vi "Pockels Cal load-Load handler.vi"(11 "Loaded pockels cal file":refnum<vi>) -> ()   [LabVIEW 2013]
uses:
  Typedefs/Which path.ctl
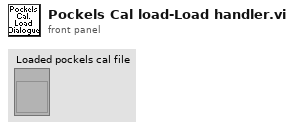
[diagram p1: front panel]
types:
  T1 = typedef "Which path.ctl" = enum16{"Configuration Files", "Calibration Files", "Images", "Setup.ini", "Loaded User profile.ini", "User's-Previous session.ini", "New user profile.ini", "Selected User profile.ini", "User profiles folder", "Power meter scaling.txt", "FOV Cal.ini"}
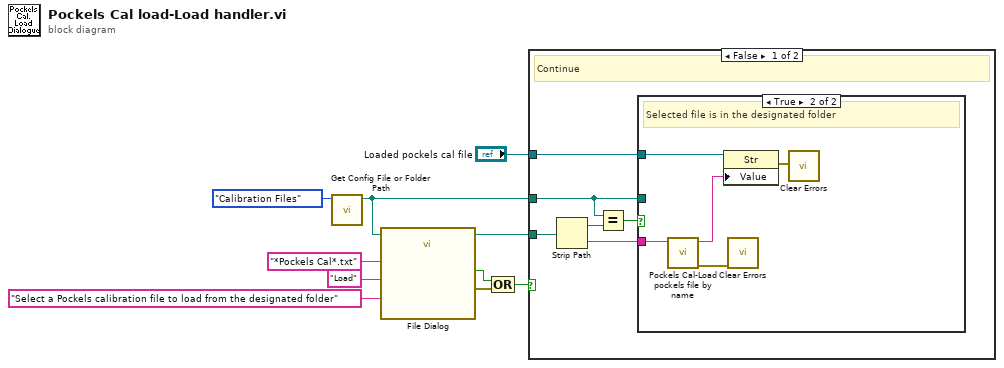
[diagram p0: block diagram]
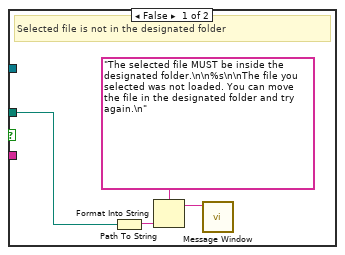
[diagram p2: hidden frame]
diagram:
  n1 = call "Get Config File or Folder Path.vi"("Which file or folder?"=Which_path."Calibration Files" ("Which file?")) -> ("File Path"=w2:path)  [unwired: 8 in, 2 out]
  n2 = call "File Dialog"("start path"=w2, "prompt"="Select a Pockels calibration file to load from the designated folder", "button label"="Load", "pattern (all files)"="*Pockels Cal*.txt") -> ("selected path"=w3:path, "cancelled"=w8:bool, "error out"=w7:errorcluster)  [unwired: 8 in, 1 out]
  n3 = Compound Arithmetic op=OR(w8, w7) -> (w6:bool)
  n4 = case shown="False" w6 {
    tunnel: w3 -> [w16 _]
    tunnel: w2 -> [w12 _]
    tunnel: "Loaded pockels cal file" -> [w11 _]
    frame False {
      # "Continue"
      n5 = Strip Path(path=w16) -> (stripped path=w14:path, name=w15:string)
      n6 = Equal?(x=w12, y=w14) -> (x = y?=w13:bool)
      n7 = case shown="True" w13 {
        tunnel: w15 -> [_ w24]
        tunnel: w12 -> [w17 _]
        tunnel: w11 -> [_ w25]
        frame False {
          # "Selected file is not in the designated folder"
          n8 = Path To String(path=w17) -> (string=w18:string)
          n9 = Format Into String(format string="The selected file MUST be inside the designated folder.\n\n%s\n\nThe file you selected was not loaded. You can move the file in the designated folder and try again.\n" ("Message string"), w18) -> (resulting string=w19:string)  [unwired: 2 in, 1 out]
          n10 = call "Message Window.vi"("Message string"=w19) -> ()  [unwired: 10 in, 1 out]
        }
        frame True {
          # "Selected file is in the designated folder"
          n11 = call "Pockels Cal-Load pockels file by name.vi"("Pockels cal file name"=w24) -> ("error out"=w21:errorcluster, "Pockels cal file name"=w23:string)  [unwired: 9 in]
          n12 = property class="Str"(reference=w25, "Value"=w23) -> (error out=w22:errorcluster)  [unwired: 1 in, 1 out]
          n13 = call <vilib>:"Clear Errors.vi"("error in (no error)"=w21) -> ()  [unwired: 6 in, 1 out]
          n14 = call <vilib>:"Clear Errors.vi"("error in (no error)"=w22) -> ()  [unwired: 6 in, 1 out]
        }
      }
    }
    frame True {
      # "Cancelled or Error"
    }
  }
